vi "Compute slopes from compensate values bis.vi"(6 "Position centre pupille (µm)\nréférence (0,0)":cluster{"X":sgl, "Y":sgl}, 7 "Dimensions":T3, 9 "Filtre":T1, 10 "Coefs (mrad/µm et mrad)":sgl[](array[numeric]), 11 "Pentes":T2) -> (2 "PentesY (mrad)":sgl[][](array[numeric]), 3 "PentesX (mrad)":sgl[][](array[numeric]))   [LabVIEW 2020]
uses:
  General dimensions definition.ctl
  Point2D.ctl
  Point2Df.ctl
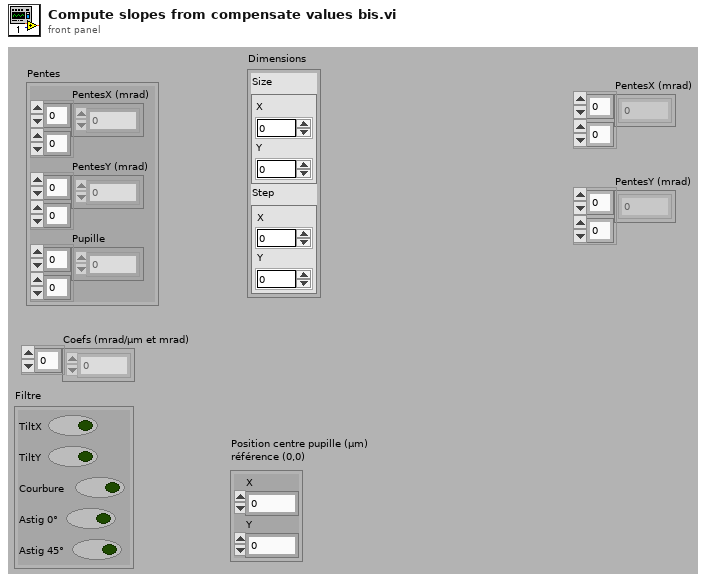
[diagram p1: front panel]
types:
  T1 = cluster{"TiltX":bool, "TiltY":bool, "Courbure":bool, "Astig 0°":bool, "Astig 45°":bool}
  T2 = cluster{"PentesX (mrad)":sgl[][], "PentesY (mrad)":sgl[][], "Pupille":i8[][]}
  T3 = typedef "General dimensions definition.ctl" = cluster{"Size":T4, "Step":T5}
  T4 = typedef "Point2D.ctl" = cluster{"X":u32, "Y":u32}
  T5 = typedef "Point2Df.ctl" = cluster{"X":sgl, "Y":sgl}
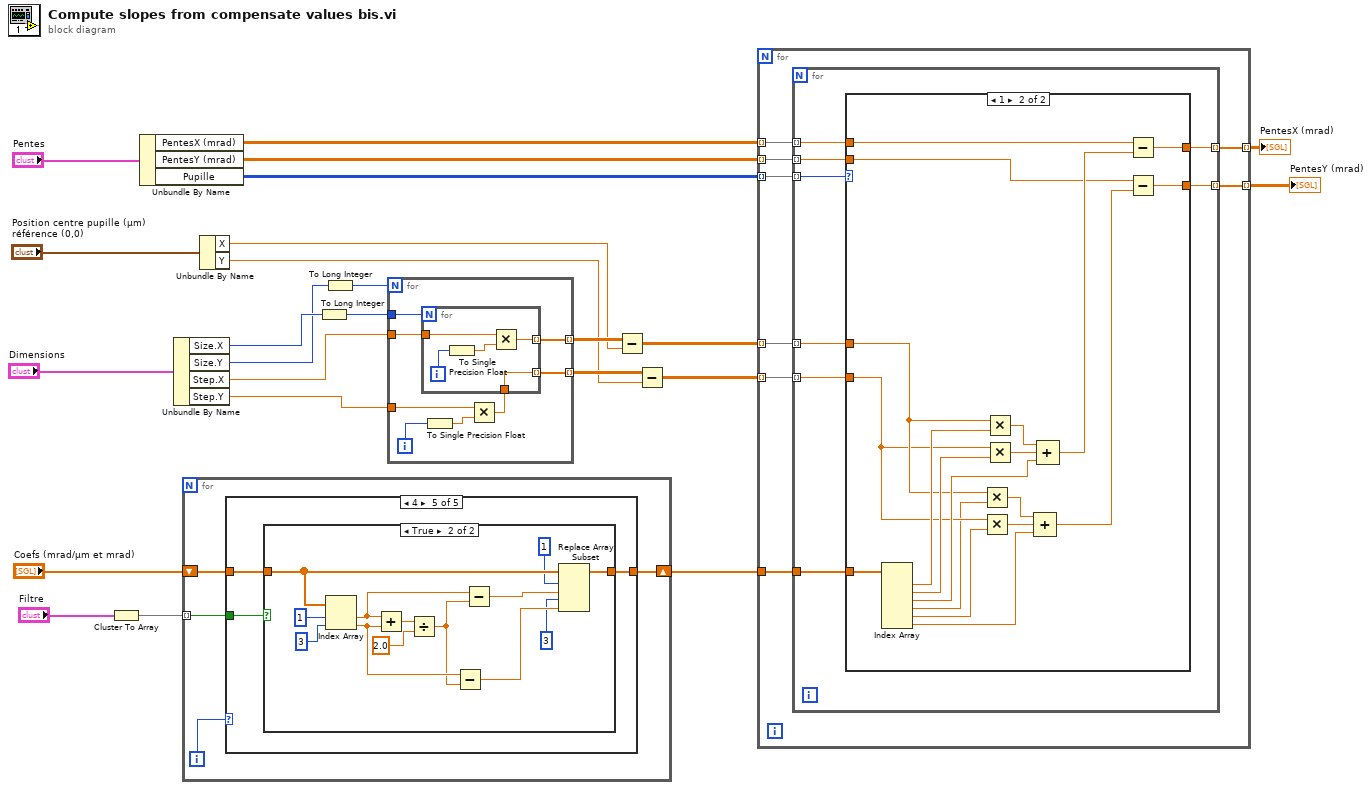
[diagram p0: block diagram]
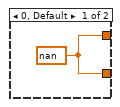
[diagram p2: hidden frame]
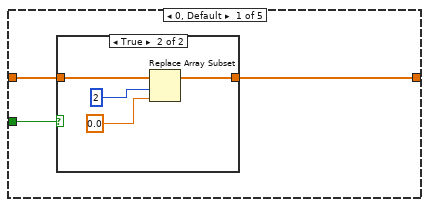
[diagram p3: hidden frame]
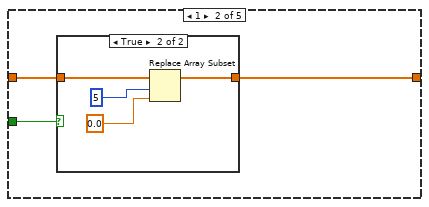
[diagram p5: hidden frame]
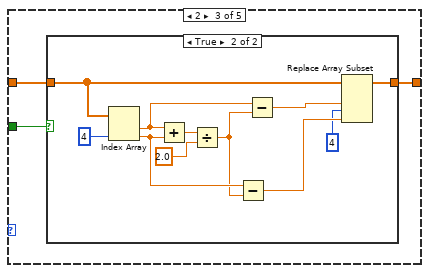
[diagram p7: hidden frame]
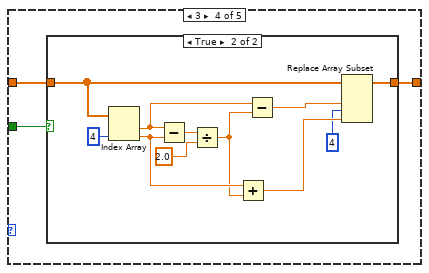
[diagram p9: hidden frame]
diagram:
  n1 = Cluster To Array(cluster="Filtre") -> (array=w16:bool[])
  n2 = Unbundle By Name("Pentes") -> ("PentesX (mrad)"=w6:sgl[][], "PentesY (mrad)"=w5:sgl[][], "Pupille"=w4:i8[][])
  n3 = Unbundle By Name("Dimensions") -> ("Size.X"=w23:u32, "Size.Y"=w20:u32, "Step.X"=w21:sgl, "Step.Y"=w18:sgl)
  n4 = for {
    tunnel: w16 -> [w28] mode=indexing
    shift-right: [w26] -> w3
    shift-left: "Coefs (mrad/µm et mrad)" -> [w27]
    i -> [w25]
    n5 = case shown="4" w25 {
      tunnel: w28 -> [w31 w39 w47 w62 w77]
      tunnel: w27 -> [w30 w38 w46 w61 w76]
      tunnel: [w29 w37 w45 w60 w75] -> w26
      frame 0, Default {
        n6 = case shown="True" w31 {
          tunnel: w30 -> [w32 w36]
          tunnel: [w32 w35] -> w29
          frame False {
          }
          frame True {
            n7 = Replace Array Subset(array=w36, new element=sgl 0.0 ("new element/subarray"), index=2) -> (w35:sgl[])
          }
        }
      }
      frame 1 {
        n8 = case shown="True" w39 {
          tunnel: w38 -> [w40 w44]
          tunnel: [w40 w43] -> w37
          frame False {
          }
          frame True {
            n9 = Replace Array Subset(array=w44, new element=sgl 0.0 ("new element/subarray"), index=5) -> (w43:sgl[])
          }
        }
      }
      frame 2 {
        n10 = case shown="True" w47 {
          tunnel: w46 -> [w48 w49]
          tunnel: [w48 w59] -> w45
          frame False {
          }
          frame True {
            n11 = Index Array(array=w49, index #2=4 ("index")) -> (element #1=w55:sgl, element #2=w54:sgl)  [unwired: 1 in]
            n12 = Add(x=w55, y=w54) -> (x+y=w57:sgl)
            n13 = Divide(x=w57, y=sgl 2.0) -> (x/y=w53:sgl)
            n14 = Subtract(x=w54, y=w53) -> (x-y=w51:sgl)
            n15 = Subtract(x=w55, y=w53) -> (x-y=w52:sgl)
            n16 = Replace Array Subset(array=w49, new element #1=w52, new element #2=w51, index #2=4 ("index")) -> (w59:sgl[])  [unwired: 1 in]
          }
        }
      }
      frame 3 {
        n17 = case shown="True" w62 {
          tunnel: w61 -> [w63 w64]
          tunnel: [w63 w74] -> w60
          frame False {
          }
          frame True {
            n18 = Index Array(array=w64, index #2=4 ("index")) -> (element #1=w70:sgl, element #2=w69:sgl)  [unwired: 1 in]
            n19 = Subtract(x=w70, y=w69) -> (x-y=w72:sgl)
            n20 = Divide(x=w72, y=sgl 2.0) -> (x/y=w68:sgl)
            n21 = Add(x=w69, y=w68) -> (x+y=w66:sgl)
            n22 = Subtract(x=w70, y=w68) -> (x-y=w67:sgl)
            n23 = Replace Array Subset(array=w64, new element #1=w67, new element #2=w66, index #2=4 ("index")) -> (w74:sgl[])  [unwired: 1 in]
          }
        }
      }
      frame 4 {
        n24 = case shown="True" w77 {
          tunnel: w76 -> [w78 w81]
          tunnel: [w78 w91] -> w75
          frame False {
          }
          frame True {
            n25 = Index Array(array=w81, index #1=1 ("index"), index #2=3 ("index")) -> (element #1=w87:sgl, element #2=w86:sgl)
            n26 = Add(x=w87, y=w86) -> (x+y=w89:sgl)
            n27 = Divide(x=w89, y=sgl 2.0) -> (x/y=w85:sgl)
            n28 = Subtract(x=w86, y=w85) -> (x-y=w83:sgl)
            n29 = Subtract(x=w87, y=w85) -> (x-y=w84:sgl)
            n30 = Replace Array Subset(array=w81, new element #1=w84, index #1=1 ("index"), new element #2=w83, index #2=3 ("index")) -> (w91:sgl[])
          }
        }
      }
    }
  }
  n31 = Unbundle By Name("Position centre pupille (µm)\nréférence (0,0)") -> ("X"=w12:sgl, "Y"=w10:sgl)
  n32 = To Long Integer(number=w23) -> (32bit integer=w22:i32)
  n33 = To Long Integer(number=w20) -> (32bit integer=w19:i32)
  n34 = for {
    N: w19 -> [_]
    tunnel: w22 -> [w99]
    tunnel: w21 -> [w98]
    tunnel: [w97] -> w14 mode=indexing
    tunnel: w18 -> [w94]
    tunnel: [w92] -> w11 mode=indexing
    i -> [w95]
    n35 = To Single Precision Float(number=w95) -> (single precision float=w96:sgl)
    n36 = Multiply(x=w94, y=w96) -> (x*y=w93:sgl)
    n37 = for {
      N: w99 -> [_]
      tunnel: w98 -> [w104]
      tunnel: [w101] -> w97 mode=indexing
      tunnel: w93 -> [w100]
      tunnel: [w100] -> w92 mode=indexing
      i -> [w103]
      n38 = To Single Precision Float(number=w103) -> (single precision float=w102:sgl)
      n39 = Multiply(x=w104, y=w102) -> (x*y=w101:sgl)
    }
  }
  n40 = Subtract(x=w14, y=w12) -> (x-y=w9:sgl[][])
  n41 = Subtract(x=w11, y=w10) -> (x-y=w8:sgl[][])
  n42 = for {
    tunnel: w9 -> [w112] mode=indexing
    tunnel: w8 -> [w111] mode=indexing
    tunnel: w6 -> [w110] mode=indexing
    tunnel: w5 -> [w109] mode=indexing
    tunnel: w4 -> [w108] mode=indexing
    tunnel: w3 -> [w107]
    tunnel: [w106] -> w2 mode=indexing
    tunnel: [w105] -> w1 mode=indexing
    n43 = for {
      tunnel: w112 -> [w116] mode=indexing
      tunnel: w111 -> [w115] mode=indexing
      tunnel: w110 -> [w119] mode=indexing
      tunnel: w109 -> [w117] mode=indexing
      tunnel: w108 -> [w120] mode=indexing
      tunnel: w107 -> [w118]
      tunnel: [w114] -> w106 mode=indexing
      tunnel: [w113] -> w105 mode=indexing
      n44 = case shown="1" w120 {
        tunnel: w119 -> [_ w134]
        tunnel: w118 -> [_ w140]
        tunnel: w117 -> [_ w132]
        tunnel: w116 -> [_ w129]
        tunnel: w115 -> [_ w128]
        tunnel: [w121 w123] -> w114
        tunnel: [w121 w122] -> w113
        frame 0, Default {
          w121 = sgl nan
        }
        frame 1 {
          n45 = Index Array(array=w140) -> (element #1=w139:sgl, element #2=w138:sgl, element #3=w135:sgl, element #4=w127:sgl, element #5=w126:sgl, element #6=w125:sgl)  [unwired: 6 in]
          n46 = Multiply(x=w129, y=w127) -> (x*y=w131:sgl)
          n47 = Multiply(x=w128, y=w126) -> (x*y=w130:sgl)
          n48 = Multiply(x=w129, y=w139) -> (x*y=w136:sgl)
          n49 = Multiply(x=w128, y=w138) -> (x*y=w137:sgl)
          n50 = Compound Arithmetic op=ADD(w131, w130, w125) -> (w124:sgl)
          n51 = Compound Arithmetic op=ADD(w136, w137, w135) -> (w133:sgl)
          n52 = Subtract(x=w134, y=w133) -> (x-y=w123:sgl)
          n53 = Subtract(x=w132, y=w124) -> (x-y=w122:sgl)
        }
      }
    }
  }
  "PentesX (mrad)" <- w2
  "PentesY (mrad)" <- w1
